vi "Current and Voltage Traces.vi"(3 "Measurement":T1) -> (0 "Current Plot":cluster{"Sequence":dbl[], "Data":dbl[]}[](array[cluster]), 1 "Voltage Plot":cluster{"Sequence":dbl[], "Data":dbl[]}[](array[cluster]))   [LabVIEW 2014]
panel:
  # "LICENSED MATERIALS – PROPERTY OF IBM\nCopyright IBM Corp. 2016,\nALL RIGHTS RESERVED"
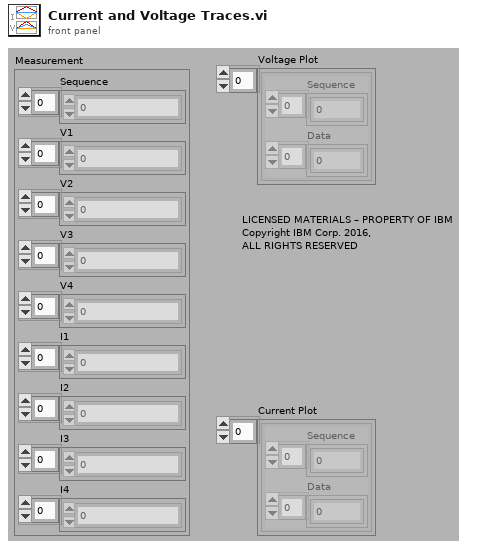
[diagram p1: front panel]
types:
  T1 = cluster{"Sequence":dbl[], "V1":dbl[], "V2":dbl[], "V3":dbl[], "V4":dbl[], "I1":dbl[], "I2":dbl[], "I3":dbl[], "I4":dbl[]}
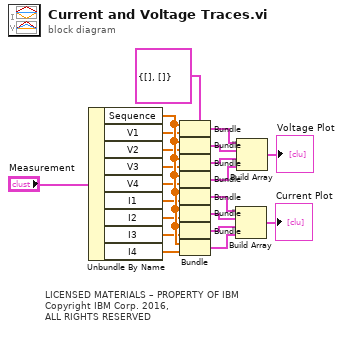
[diagram p0: block diagram]
diagram:
  w21 = cluster{"Sequence":dbl[], "Data":dbl[]} {"Sequence"=[], "Data"=[]} ("Cluster")
  # "LICENSED MATERIALS – PROPERTY OF IBM\nCopyright IBM Corp. 2016,\nALL RIGHTS RESERVED"
  n1 = Unbundle By Name("Measurement") -> ("Sequence"=w19:dbl[], "V1"=w18:dbl[], "V2"=w17:dbl[], "V3"=w16:dbl[], "V4"=w15:dbl[], "I1"=w14:dbl[], "I2"=w13:dbl[], "I3"=w12:dbl[], "I4"=w11:dbl[])
  n2 = Bundle ("V1")(cluster=w21, "Sequence"=w19, "Data"=w18) -> (w10:cluster{"Sequence":dbl[], "Data":dbl[]})
  n3 = Bundle ("V2")(cluster=w21, "Sequence"=w19, "Data"=w17) -> (w9:cluster{"Sequence":dbl[], "Data":dbl[]})
  n4 = Bundle ("V3")(cluster=w21, "Sequence"=w19, "Data"=w16) -> (w8:cluster{"Sequence":dbl[], "Data":dbl[]})
  n5 = Bundle ("V4")(cluster=w21, "Sequence"=w19, "Data"=w15) -> (w7:cluster{"Sequence":dbl[], "Data":dbl[]})
  n6 = Bundle ("I1")(cluster=w21, "Sequence"=w19, "Data"=w14) -> (w6:cluster{"Sequence":dbl[], "Data":dbl[]})
  n7 = Bundle ("I2")(cluster=w21, "Sequence"=w19, "Data"=w13) -> (w5:cluster{"Sequence":dbl[], "Data":dbl[]})
  n8 = Bundle ("I3")(cluster=w21, "Sequence"=w19, "Data"=w12) -> (w4:cluster{"Sequence":dbl[], "Data":dbl[]})
  n9 = Bundle ("I4")(cluster=w21, "Sequence"=w19, "Data"=w11) -> (w3:cluster{"Sequence":dbl[], "Data":dbl[]})
  n10 = Build Array(w6, w5, w4, w3) -> (→"Current Plot":cluster{"Sequence":dbl[], "Data":dbl[]}[])
  n11 = Build Array(w10, w9, w8, w7) -> (→"Voltage Plot":cluster{"Sequence":dbl[], "Data":dbl[]}[])
